vi "菜单-另存为.vi"(8 "error in (no error)":errorcluster caption="错误输入（无错误）", 11 "程序响应 输入":refnum<class "程序响应.lvclass">) -> (0 "error out":errorcluster caption="错误输出", 3 "程序响应 输出":refnum<class "程序响应.lvclass">)   [LabVIEW 2018, in "程序响应.lvlib" / "程序响应.lvclass"]
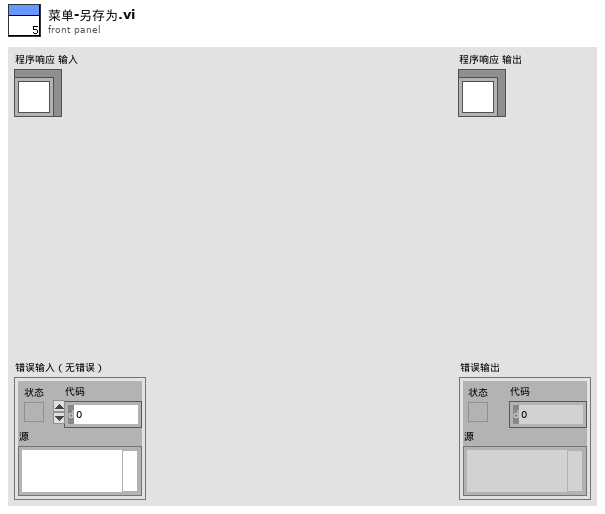
[diagram p1: front panel]
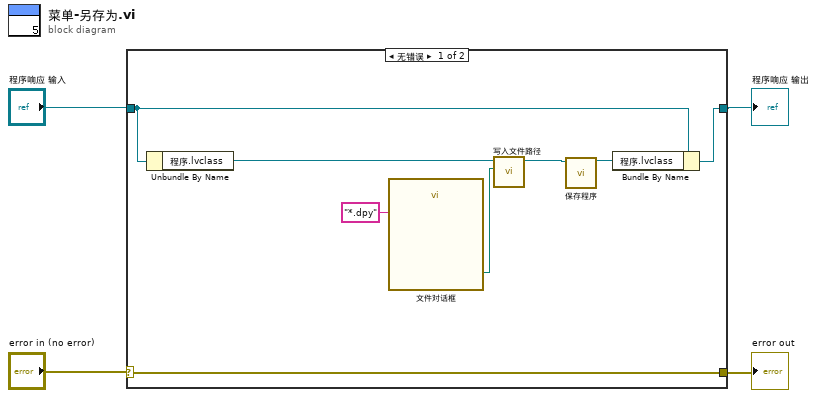
[diagram p0: block diagram]
diagram:
  n1 = case shown="无错误" "error in (no error)" {
    selector: "error in (no error)" -> [w12 w14]
    tunnel: [w12 w14] -> w1
    tunnel: [w8 w13] -> w4
    tunnel: "程序响应 输入" -> [w9 w13]
    frame No Error {
      n2 = Unbundle By Name(w9) -> ("程序.lvclass"=w11:refnum<class "程序.lvclass">)
      n3 = call "文件对话框"("pattern (all files)"="*.dpy" ("pattern label")) -> ("selected path"=w6:path)  [unwired: 11 in, 3 out]
      n4 = call-dynamic "写入文件路径.vi"("文件路径"=w6, "程序输入"=w11) -> ("程序输出"=w7:refnum<class "程序.lvclass">)  [unwired: 8 in, 1 out]
      n5 = call-dynamic "保存程序.vi"("程序 输入"=w7) -> ("程序 输出"=w10:refnum<class "程序.lvclass">)  [unwired: 9 in, 1 out]
      n6 = Bundle By Name(cluster=w9, "程序.lvclass"=w10) -> (w8:refnum<class "程序响应.lvclass">)
    }
    frame Error {
    }
  }
  "error out" <- w1
  "程序响应 输出" <- w4
